vi "rd_getColumnProperty.vi"(8 "error in (no error)":errorcluster, 9 "property":T3(ring), 10 "channel index":u32, 11 "Excel refnum":T2) -> (0 "error out":errorcluster, 1 "column Length":u64, 2 "string property":string, 3 "Excel refnum out":T2, 4 "Column DataType":T1)   [LabVIEW 2017, in "NI_ExcelFile.lvlib"]
uses:
  <vilib>/express/express shared/NI_ExcelFile/NI_ExcelFile.lvlib
  <vilib>/express/express shared/NI_ExcelFile/Ctrls/ExcelRefnum.ctl
  <vilib>/express/express shared/NI_ExcelFile/Ctrls/MainData.ctl
  <vilib>/express/express shared/NI_ExcelFile/Ctrls/StreamMode.ctl
  <vilib>/express/express shared/NI_ExcelFile/Ctrls/TimeColumnMode.ctl
  <vilib>/express/express shared/NI_ExcelFile/Ctrls/FileAttribute.ctl
  <vilib>/express/express shared/NI_ExcelFile/Ctrls/Columns.ctl
  <vilib>/express/express shared/NI_ExcelFile/Ctrls/ColumnInfo.ctl
  <vilib>/express/express shared/NI_ExcelFile/Ctrls/DataType.ctl
  <vilib>/express/express shared/NI_ExcelFile/Ctrls/wd_recordInfo.ctl
  <vilib>/express/express shared/NI_ExcelFile/Ctrls/disk_TemplateFile.ctl
  <vilib>/express/express shared/NI_ExcelFile/Ctrls/meta_file.ctl
  <vilib>/express/express shared/NI_ExcelFile/Ctrls/meta_Block.ctl
  <vilib>/express/express shared/NI_ExcelFile/Ctrls/meta_BlockType.ctl
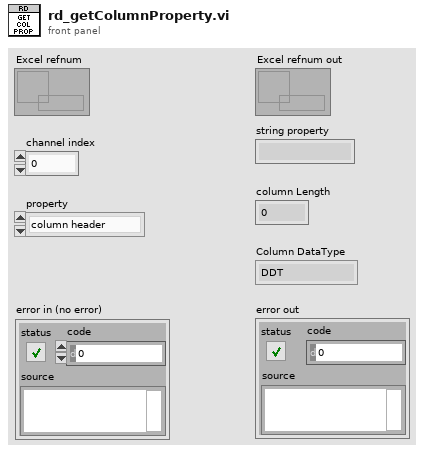
[diagram p1: front panel]
types:
  T1 = typedef "NI_ExcelFile.lvlib/DataType.ctl" = enum16{"DDT", "WFM", "Array of STR", "Array of DBL", "Array of I8", "Array of I16", "Array of I32", "Array of I64", "Array of SGL", "Array of U8", "Array of U16", "Array of U32", "Array of U64", "Array of Time"}
  T2 = typedef "NI_ExcelFile.lvlib/ExcelRefnum.ctl" = refnum<data-value>
  T3 = enum16{"column header", "column format", "column datatype", "column length"}
  T4 = typedef "NI_ExcelFile.lvlib/MainData.ctl" = cluster{"TargetFile":path, "StreamMode":T5, "Append?":bool, "ChunkSize":u64, "TimeColumnMode":T6, "TimestampFormat":string, "AbsoluteTime?":bool, "FileAttribute ":T7, "Column":T8, "FileRef":refnum<k1>, "MemoryRef":refnum<data-value>[], "RecordInfo":T10[], " ChannelPreviousInfo":u32[], "ChannelFirstRecord":u32[], "PredefinedFormattedValueLength":i64, "DiskTemplate":T11}
  T5 = typedef "NI_ExcelFile.lvlib/StreamMode.ctl" = enum16{"File", "Memory"}
  T6 = typedef "NI_ExcelFile.lvlib/TimeColumnMode.ctl" = enum16{"Empty", "OnePerCh", "One"}
  T7 = typedef "NI_ExcelFile.lvlib/FileAttribute.ctl" = cluster{"Creator":string, "Title":string, "SheetName":string}
  T8 = typedef "NI_ExcelFile.lvlib/Columns.ctl" = T9[]
  T9 = typedef "NI_ExcelFile.lvlib/ColumnInfo.ctl" = cluster{"Header":string, "Format":string, "DataType":T1, "Length":u64}
  T10 = typedef "NI_ExcelFile.lvlib/wd_recordInfo.ctl" = cluster{"ChannelIndex":u32, "StartIndex":u64, "Length":u64, "Previous":i32, "Next":i32}
  T11 = typedef "NI_ExcelFile.lvlib/disk_TemplateFile.ctl" = cluster{"XMLRef":refnum<file>[], "ZipPath":path, "MetaFile":T12, "TempFolder":path}
  T12 = typedef "NI_ExcelFile.lvlib/meta_file.ctl" = cluster{"Ref":refnum<file>, "NextRow":i32, "NextPosition":i64, "Block":T13[]}
  T13 = typedef "NI_ExcelFile.lvlib/meta_Block.ctl" = cluster{"Version":u16, "Type":T14, "Length":i32, "Data":string}
  T14 = typedef "NI_ExcelFile.lvlib/meta_BlockType.ctl" = enum16{"NITag", "File", "Column"}
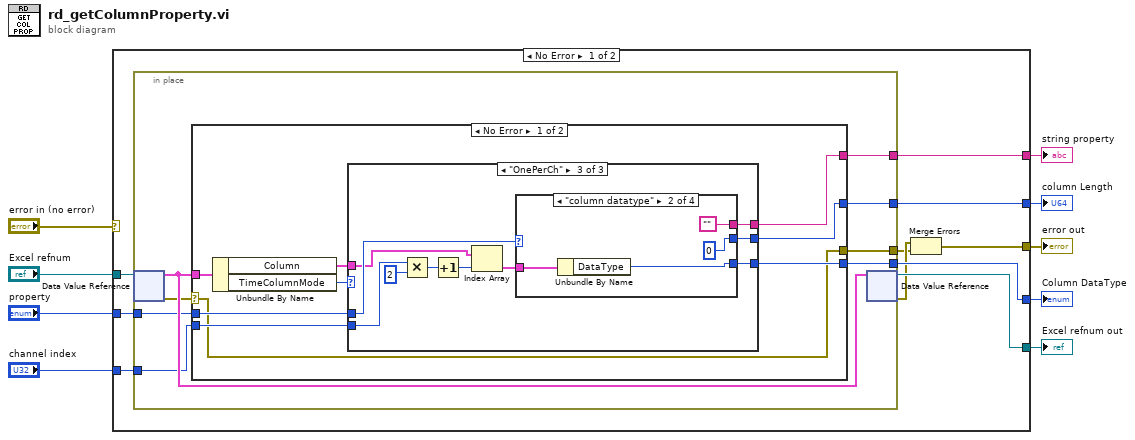
[diagram p0: block diagram]
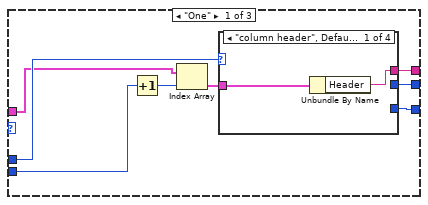
[diagram p2: hidden frame]
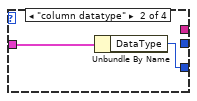
[diagram p3: hidden frame]
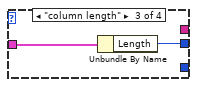
[diagram p4: hidden frame]
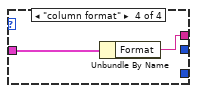
[diagram p5: hidden frame]
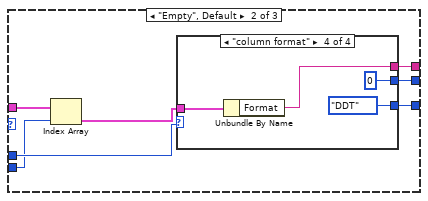
[diagram p6: hidden frame]
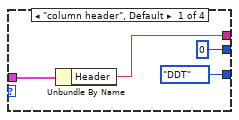
[diagram p7: hidden frame]
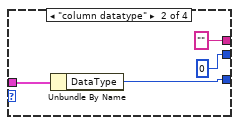
[diagram p8: hidden frame]
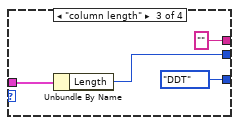
[diagram p9: hidden frame]
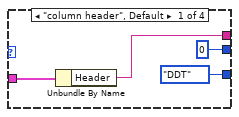
[diagram p10: hidden frame]
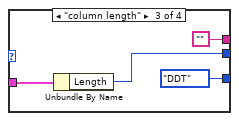
[diagram p11: hidden frame]
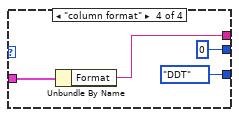
[diagram p12: hidden frame]
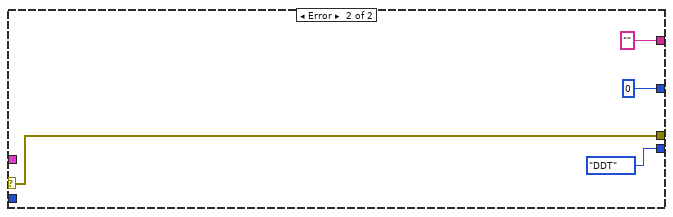
[diagram p13: hidden frame]
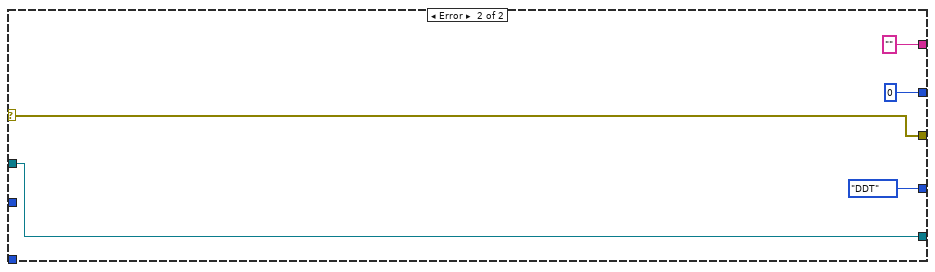
[diagram p14: hidden frame]
diagram:
  n1 = case shown="No Error" "error in (no error)" {
    selector: "error in (no error)" -> [_ w110]
    tunnel: "Excel refnum" -> [w19 w109]
    tunnel: "property" -> [w18 _]
    tunnel: "channel index" -> [w17 _]
    tunnel: [w16 "" ("Format")] -> w6
    tunnel: [w15 u64 0 ("Length")] -> w5
    tunnel: [w14 w109] -> w4
    tunnel: [w10 w110] -> w2
    tunnel: [w13 DataType."DDT" ("DataType")] -> w1
    frame No Error {
      n2 = in-place {
        in-place-border: w18 -> [w26]
        in-place-border: w17 -> [w25]
        in-place-border: [w24] -> w16
        in-place-border: [w23] -> w15
        in-place-border: [w22] -> w13
        in-place-border: [w20] -> w11
        n3 = in-place-dvr #1(w19) -> (w27:T4, w21:errorcluster)
        n4 = case shown="No Error" w21 {
          selector: w21 -> [w28 w102]
          tunnel: w27 -> [w36 _]
          tunnel: w26 -> [w35 _]
          tunnel: w25 -> [w33 _]
          tunnel: [w32 "" ("Format")] -> w24
          tunnel: [w31 u64 0 ("Length")] -> w23
          tunnel: [w29 DataType."DDT" ("DataType")] -> w22
          tunnel: [w28 w102] -> w20
          frame No Error {
            n5 = Unbundle By Name(w36) -> ("Column"=w34:T8, "TimeColumnMode"=w30:T6)
            n6 = case shown="\"OnePerCh\"" w30 {
              tunnel: w35 -> [w44 w59 w85]
              tunnel: w34 -> [w43 w58 w84]
              tunnel: w33 -> [w39 w57 w80]
              tunnel: [w41 w55 w82] -> w32
              tunnel: [w40 w54 w81] -> w31
              tunnel: [w37 w53 w76] -> w29
              frame "One" {
                n7 = Increment(x=w39) -> (x+1=w38:u32)
                n8 = Index Array(array=w43, index=w38) -> (element=w42:T9)
                n9 = case shown="\"column header\", Default" w44 {
                  tunnel: w42 -> [w46 w48 w50 w52]
                  tunnel: [w45 _ _ w51] -> w41
                  tunnel: [_ _ w49 _] -> w40
                  tunnel: [_ w47 _ _] -> w37
                  frame "column header", Default {
                    n10 = Unbundle By Name(w46) -> ("Header"=w45:string)
                  }
                  frame "column datatype" {
                    n11 = Unbundle By Name(w48) -> ("DataType"=w47:T1)
                  }
                  frame "column length" {
                    n12 = Unbundle By Name(w50) -> ("Length"=w49:u64)
                  }
                  frame "column format" {
                    n13 = Unbundle By Name(w52) -> ("Format"=w51:string)
                  }
                }
              }
              frame "Empty", Default {
                n14 = Index Array(array=w58, index=w57) -> (element=w56:T9)
                n15 = case shown="\"column format\"" w59 {
                  tunnel: w56 -> [w63 w67 w71 w75]
                  tunnel: [w62 "" ("Format") "" ("Format") w74] -> w55
                  tunnel: [u64 0 ("Length") u64 0 ("Length") w70 u64 0 ("Length")] -> w54
                  tunnel: [DataType."DDT" ("DataType") w66 DataType."DDT" ("DataType") DataType."DDT" ("DataType")] -> w53
                  frame "column header", Default {
                    n16 = Unbundle By Name(w63) -> ("Header"=w62:string)
                  }
                  frame "column datatype" {
                    n17 = Unbundle By Name(w67) -> ("DataType"=w66:T1)
                  }
                  frame "column length" {
                    n18 = Unbundle By Name(w71) -> ("Length"=w70:u64)
                  }
                  frame "column format" {
                    n19 = Unbundle By Name(w75) -> ("Format"=w74:string)
                  }
                }
              }
              frame "OnePerCh" {
                n20 = Multiply(x=w80, y=2) -> (x*y=w78:u32)
                n21 = Increment(x=w78) -> (x+1=w77:u32)
                n22 = Index Array(array=w84, index=w77) -> (element=w83:T9)
                n23 = case shown="\"column datatype\"" w85 {
                  tunnel: w83 -> [w89 w93 w97 w101]
                  tunnel: [w88 "" "" ("Format") w100] -> w82
                  tunnel: [u64 0 ("Length") u64 0 ("Length") w96 u64 0 ("Length")] -> w81
                  tunnel: [DataType."DDT" ("DataType") w92 DataType."DDT" ("DataType") DataType."DDT" ("DataType")] -> w76
                  frame "column header", Default {
                    n24 = Unbundle By Name(w89) -> ("Header"=w88:string)
                  }
                  frame "column datatype" {
                    n25 = Unbundle By Name(w93) -> ("DataType"=w92:T1)
                  }
                  frame "column length" {
                    n26 = Unbundle By Name(w97) -> ("Length"=w96:u64)
                  }
                  frame "column format" {
                    n27 = Unbundle By Name(w101) -> ("Format"=w100:string)
                  }
                }
              }
            }
          }
          frame Error {
          }
        }
        n28 = in-place-dvr #1(w27) -> (w14:T2, w12:errorcluster)
      }
      n29 = Merge Errors(w12, w11) -> (w10:errorcluster)
    }
    frame Error {
    }
  }
  "string property" <- w6
  "column Length" <- w5
  "Excel refnum out" <- w4
  "Column DataType" <- w1
  "error out" <- w2
